vi "Log Event.vi"(8 "error in":errorcluster, 10 "Event Text":string, 11 "Imp Series Actor in":refnum<class "Imponator Series Actor.lvclass">) -> (0 "error out":errorcluster, 3 "Imp Series Actor out":refnum<class "Imponator Series Actor.lvclass">)   [LabVIEW 2024, in "Imponator Series Actor.lvlib" / "Imponator Series Actor.lvclass"]
uses:
  gitlab/imponator-series-actor/Imponator Series Actor/Imponator Series Actor/Imponator Series Actor.lvclass
  gitlab/imponator-series-actor/Imponator Series Actor/Imponator Series Actor/Imponator Series Actor.lvclass/Imponator Series Actor.ctl
  ISeries UI Actor/ISeries UI Actor Messages/Log Event Msg/Log Event Msg.lvclass
  Series Actor.lvclass
  gitlab/imponator-series-actor/Imponator Series Actor/Imponator Series Actor/Nested Actors Series.ctl
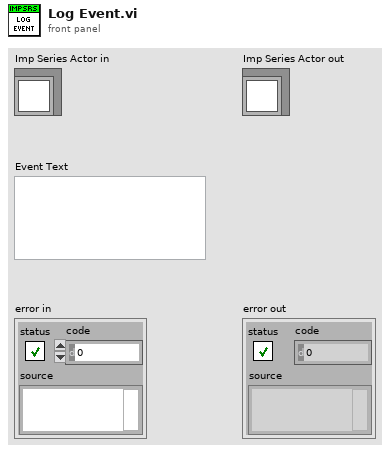
[diagram p1: front panel]
types:
  T1 = typedef "Nested Actors Series.ctl" = enum16{"GUI", "Data Logger", "Controller", "MCUs"}
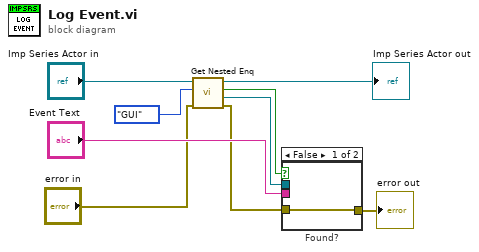
[diagram p0: block diagram]
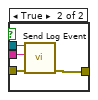
[diagram p2: hidden frame]
diagram:
  n1 = call "Get Nested Enq.vi"("error in"="error in", "Ident"=Nested_Actors_Series."GUI", "Series Actor in"="Imp Series Actor in") -> ("error out"=w3:errorcluster, "Enq"=w1:refnum<class "Message Enqueuer.lvclass">, "Found?"=w2:bool, "Series Actor out"=→"Imp Series Actor out":refnum<class "Imponator Series Actor.lvclass">)  [unwired: 5 in]
  n2 = case "Found?" shown="False" w2 {
    tunnel: "Event Text" -> [_ w14]
    tunnel: [w10 w13] -> w7
    tunnel: w3 -> [w10 w12]
    tunnel: w1 -> [_ w11]
    frame False {
    }
    frame True {
      n3 = call "Send Log Event.vi"("error in (no error)"=w12, "Event Text"=w14, "Message Enqueuer"=w11) -> ("error out"=w13:errorcluster)  [unwired: 7 in, 1 out]
    }
  }
  "error out" <- w7
